vi "ProcessBufferUpdates.vi"(11 "MockHPILCSettings":T1={"ModbusRxDataFIFO"="MockbusPort2RxFIFO", "ModbusTxDataFIFO"="ModbusPort2TxInternalFIFO", "BufferUpdateFIFO"="MockHPILCCommand", "Code17Memory"="MockHPILCCode17", "Code18Memory"="MockHPILCCode18", "Code65Memory"="MockHPILCCode65", "Code66Memory"="MockHPILCCode66", "Code67Memory"="MockHPILCCode67", "Code72Memory"="MockHPILCCode72", "Code80Memory"="MockHPILCCode80", "Code110Memory"="MockHPILCCode110"}) -> ()   [LabVIEW 2016, in "FPGAMockMDILC.lvlib"]
uses:
  FPGAMockMDILC.lvlib
  <vilib>/rvi/DataTransferAndStorage/Container/XNode/niFpgaContainer.xnode
  <vilib>/rvi/FIFO/Fifo_Resource/niFpgaFifoEmulationRefIn.vi
  <vilib>/rvi/Memory/Memory_Emulation/niFpgaMemoryEmulationRefIn.vi
  DataTypes/MockHPILCSettings.ctl
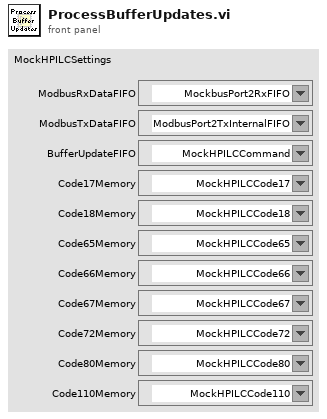
[diagram p1: front panel]
types:
  T1 = typedef "FPGAMockMDILC.lvlib/MockHPILCSettings.ctl" = cluster{"ModbusRxDataFIFO":refnum<k21>, "ModbusTxDataFIFO":refnum<k21>, "BufferUpdateFIFO":refnum<k21>, "Code17Memory":refnum<k21>, "Code18Memory":refnum<k21>, "Code65Memory":refnum<k21>, "Code66Memory":refnum<k21>, "Code67Memory":refnum<k21>, "Code72Memory":refnum<k21>, "Code80Memory":refnum<k21>, "Code110Memory":refnum<k21>}
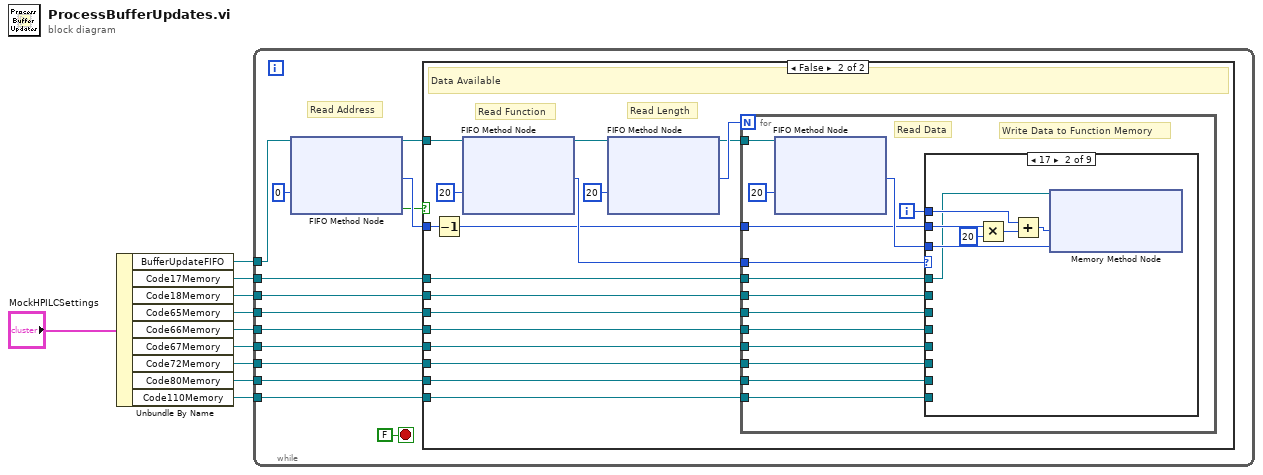
[diagram p0: block diagram]
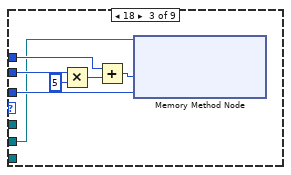
[diagram p4: hidden frame]
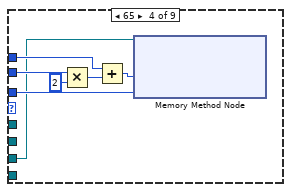
[diagram p5: hidden frame]
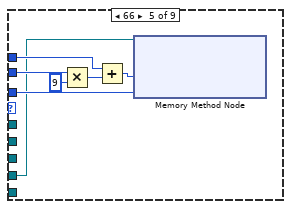
[diagram p6: hidden frame]
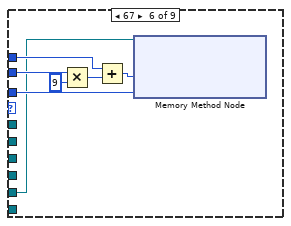
[diagram p7: hidden frame]
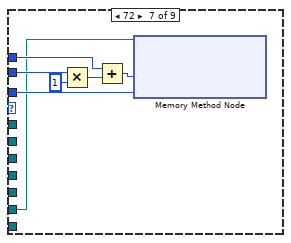
[diagram p8: hidden frame]
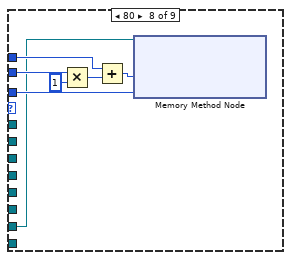
[diagram p9: hidden frame]
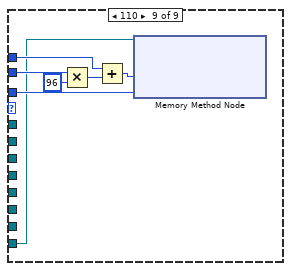
[diagram p10: hidden frame]
diagram:
  n1 = Unbundle By Name("MockHPILCSettings") -> ("BufferUpdateFIFO"=w9:refnum<k21>, "Code17Memory"=w8:refnum<k21>, "Code18Memory"=w7:refnum<k21>, "Code65Memory"=w6:refnum<k21>, "Code66Memory"=w5:refnum<k21>, "Code67Memory"=w4:refnum<k21>, "Code72Memory"=w3:refnum<k21>, "Code80Memory"=w2:refnum<k21>, "Code110Memory"=w1:refnum<k21>)
  n2 = while {
    tunnel: w9 -> [w19]
    tunnel: w8 -> [w18]
    tunnel: w7 -> [w17]
    tunnel: w6 -> [w16]
    tunnel: w5 -> [w15]
    tunnel: w4 -> [w14]
    tunnel: w3 -> [w13]
    tunnel: w2 -> [w12]
    tunnel: w1 -> [w11]
    stop <- FALSE stop-if-true
    # "Read Address"
    n3 = xnode ("FIFO Method Node")("Timeout"=0, "FIFO In"=w19) -> ("Element"=w23:u8, "Timed Out?"=w21:bool, "FIFO Out"=w24:refnum<k21>)
    n4 = case shown="False" w21 {
      tunnel: w24 -> [_ w40]
      tunnel: w23 -> [_ w36]
      tunnel: w18 -> [_ w32]
      tunnel: w17 -> [_ w31]
      tunnel: w16 -> [_ w30]
      tunnel: w15 -> [_ w29]
      tunnel: w14 -> [_ w28]
      tunnel: w13 -> [_ w27]
      tunnel: w12 -> [_ w26]
      tunnel: w11 -> [_ w25]
      frame True {
        # "No Data Available"
      }
      frame False {
        # "Read Length"
        # "Read Function"
        # "Data Available"
        n5 = Decrement(x=w36) -> (x-1=w35:u8)
        n6 = xnode ("FIFO Method Node")("Timeout"=20, "FIFO In"=w40) -> ("Element"=w37:u8, "FIFO Out"=w39:refnum<k21>)  [unwired: 1 out]
        n7 = xnode ("FIFO Method Node")("Timeout"=20, "FIFO In"=w39) -> ("Element"=w41:u8, "FIFO Out"=w38:refnum<k21>)  [unwired: 1 out]
        n8 = for {
          N: w41 -> [_]
          tunnel: w38 -> [w55]
          tunnel: w37 -> [w54]
          tunnel: w35 -> [w52]
          tunnel: w32 -> [w49]
          tunnel: w31 -> [w48]
          tunnel: w30 -> [w47]
          tunnel: w29 -> [w46]
          tunnel: w28 -> [w45]
          tunnel: w27 -> [w44]
          tunnel: w26 -> [w43]
          tunnel: w25 -> [w42]
          i -> [w50]
          # "Write Data to Function Memory"
          # "Read Data"
          n9 = xnode ("FIFO Method Node")("Timeout"=20, "FIFO In"=w55) -> ("Element"=w53:u8)  [unwired: 2 out]
          n10 = case shown="17" w54 {
            tunnel: w53 -> [_ w62 w69 w76 w83 w90 w97 w104 w111]
            tunnel: w52 -> [_ w61 w68 w75 w82 w89 w96 w103 w110]
            tunnel: w50 -> [_ w57 w64 w71 w78 w85 w92 w99 w106]
            tunnel: w49 -> [_ w56 _ _ _ _ _ _ _]
            tunnel: w48 -> [_ _ w63 _ _ _ _ _ _]
            tunnel: w47 -> [_ _ _ w70 _ _ _ _ _]
            tunnel: w46 -> [_ _ _ _ w77 _ _ _ _]
            tunnel: w45 -> [_ _ _ _ _ w84 _ _ _]
            tunnel: w44 -> [_ _ _ _ _ _ w91 _ _]
            tunnel: w43 -> [_ _ _ _ _ _ _ w98 _]
            tunnel: w42 -> [_ _ _ _ _ _ _ _ w105]
            frame 0, Default {
            }
            frame 17 {
              n11 = Multiply(x=w61, y=u8 20) -> (x*y=w59:u8)
              n12 = Add(x=w57, y=w59) -> (x+y=w58:i32)
              n13 = xnode ("Memory Method Node")("Address"=w58, "Data"=w62, "Memory In"=w56) -> ()  [unwired: 1 out]
            }
            frame 18 {
              n14 = Multiply(x=w68, y=u8 5) -> (x*y=w66:u8)
              n15 = Add(x=w64, y=w66) -> (x+y=w65:i32)
              n16 = xnode ("Memory Method Node")("Address"=w65, "Data"=w69, "Memory In"=w63) -> ()  [unwired: 1 out]
            }
            frame 65 {
              n17 = Multiply(x=w75, y=u8 2) -> (x*y=w73:u8)
              n18 = Add(x=w71, y=w73) -> (x+y=w72:i32)
              n19 = xnode ("Memory Method Node")("Address"=w72, "Data"=w76, "Memory In"=w70) -> ()  [unwired: 1 out]
            }
            frame 66 {
              n20 = Multiply(x=w82, y=u8 9) -> (x*y=w80:u8)
              n21 = Add(x=w78, y=w80) -> (x+y=w79:i32)
              n22 = xnode ("Memory Method Node")("Address"=w79, "Data"=w83, "Memory In"=w77) -> ()  [unwired: 1 out]
            }
            frame 67 {
              n23 = Multiply(x=w89, y=u8 9) -> (x*y=w87:u8)
              n24 = Add(x=w85, y=w87) -> (x+y=w86:i32)
              n25 = xnode ("Memory Method Node")("Address"=w86, "Data"=w90, "Memory In"=w84) -> ()  [unwired: 1 out]
            }
            frame 72 {
              n26 = Multiply(x=w96, y=u8 1) -> (x*y=w94:u8)
              n27 = Add(x=w92, y=w94) -> (x+y=w93:i32)
              n28 = xnode ("Memory Method Node")("Address"=w93, "Data"=w97, "Memory In"=w91) -> ()  [unwired: 1 out]
            }
            frame 80 {
              n29 = Multiply(x=w103, y=u8 1) -> (x*y=w101:u8)
              n30 = Add(x=w99, y=w101) -> (x+y=w100:i32)
              n31 = xnode ("Memory Method Node")("Address"=w100, "Data"=w104, "Memory In"=w98) -> ()  [unwired: 1 out]
            }
            frame 110 {
              n32 = Multiply(x=w110, y=u8 96) -> (x*y=w108:u8)
              n33 = Add(x=w106, y=w108) -> (x+y=w107:i32)
              n34 = xnode ("Memory Method Node")("Address"=w107, "Data"=w111, "Memory In"=w105) -> ()  [unwired: 1 out]
            }
          }
        }
      }
    }
  }
